vi "Determine Active DTCs and Timestamps.vi"(9 "current time":timestamp, 10 "Previous Changed DTCs":T2[](array[typedef]), 11 "current DTCs":T1[](array[typedef])) -> (3 "Active DTCs":T2[](array[typedef]))   [LabVIEW 2015, in "Diagnostics Addon Engine.lvlib"]
doc: "Does this:\n- if DTC is no longer active, delete it\n- if DTC is new, add it, if it has been there before, update it to latest data\n- Sort DTCs - newest first"
uses:
  Diagnostics Addon Engine.lvlib
  Shared/Types/DTC.Info.ctl
  <vilib>/Automotive Diagnostic Command Set/Diagnostic Protocols.llb/Diagnostic Trouble Code.ctl
  Shared/Diagnostics Addon Shared.lvlib
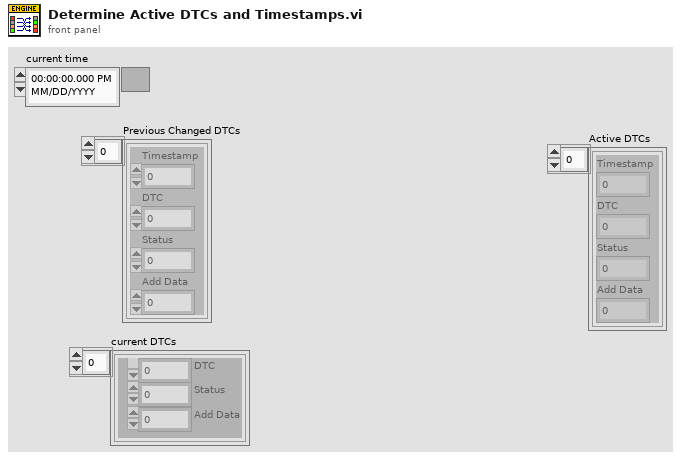
[diagram p1: front panel]
types:
  T1 = typedef "Diagnostic Trouble Code.ctl" = cluster{"DTC":u32, "Status":u32, "Add Data":u32}
  T2 = typedef "Diagnostics Addon Shared.lvlib/DTC.Info.ctl" = cluster{"Timestamp":dbl, "DTC":dbl, "Status":dbl, "Add Data":dbl}
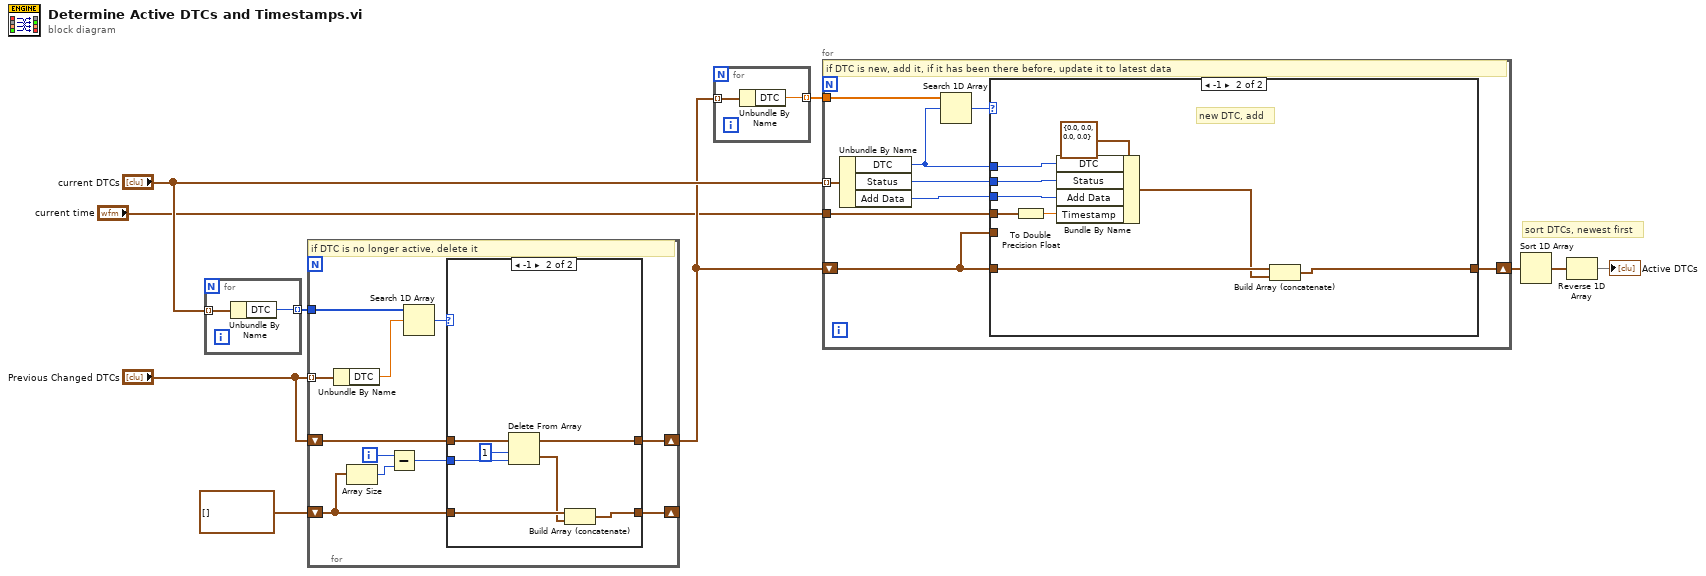
[diagram p0: block diagram]
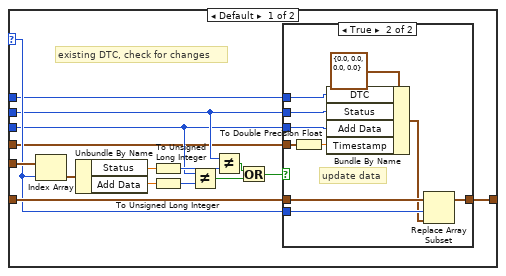
[diagram p3: hidden frame]
diagram:
  # "sort DTCs, newest first"
  n1 = for {
    tunnel: "current DTCs" -> [w12] mode=indexing
    tunnel: [w11] -> w8 mode=indexing
    n2 = Unbundle By Name(w12) -> ("DTC"=w11:u32)
  }
  n3 = for {
    tunnel: "Previous Changed DTCs" -> [w21] mode=indexing
    tunnel: w8 -> [w23]
    shift-right: [w19] -> w3
    shift-left: "Previous Changed DTCs" -> [w20]
    shift-right: [w16] -> _
    shift-left: T2[] [] ("Previous Changed DTCs") -> [w15]
    i -> [w17]
    # "if DTC is no longer active, delete it"
    n4 = Unbundle By Name(w21) -> ("DTC"=w18:dbl)
    n5 = Array Size(array=w15) -> (size(s)=w13:i32)
    n6 = Subtract(x=w17, y=w13) -> (x-y=w14:i32)
    n7 = Search 1D Array(1D array=w23, element=w18) -> (index of element=w22:i32)  [unwired: 1 in]
    n8 = case shown="-1" w22 {
      tunnel: w20 -> [w25 w32]
      tunnel: [w25 w31] -> w19
      tunnel: w14 -> [_ w30]
      tunnel: [w24 w26] -> w16
      tunnel: w15 -> [w24 w28]
      frame Default {
      }
      frame -1 {
        n9 = Delete From Array(array=w32, length=1, index=w30) -> (deleted portion=w27:T2[], array with subset deleted=w31:T2[])
        n10 = Build Array (concatenate)(w28, w27) -> (w26:T2[])
      }
    }
  }
  n11 = for {
    tunnel: w3 -> [w34] mode=indexing
    tunnel: [w33] -> w9 mode=indexing
    n12 = Unbundle By Name(w34) -> ("DTC"=w33:dbl)
  }
  n13 = for {
    tunnel: "current DTCs" -> [w41] mode=indexing
    tunnel: w9 -> [w43]
    shift-right: [w40] -> w2
    shift-left: w3 -> [w35]
    tunnel: "current time" -> [w39]
    # "if DTC is new, add it, if it has been there before, update it to latest data"
    n14 = Unbundle By Name(w41) -> ("DTC"=w37:u32, "Status"=w38:u32, "Add Data"=w36:u32)
    n15 = Search 1D Array(1D array=w43, element=w37) -> (index of element=w42:i32)  [unwired: 1 in]
    n16 = case shown="-1" w42 {
      selector: w42 -> [w49 _]
      tunnel: w35 -> [w50 w79]
      tunnel: [w48 w78] -> w40
      tunnel: w39 -> [w44 w73]
      tunnel: w38 -> [w46 w76]
      tunnel: w37 -> [w47 w75]
      tunnel: w36 -> [w45 w74]
      tunnel: w35 -> [w59 _]
      frame Default {
        # "existing DTC, check for changes"
        n17 = Index Array(array=w59, index=w49) -> (element=w58:T2)
        n18 = Unbundle By Name(w58) -> ("Status"=w57:dbl, "Add Data"=w56:dbl)
        n19 = To Unsigned Long Integer(number=w57) -> (unsigned 32bit integer=w55:u32)
        n20 = To Unsigned Long Integer(number=w56) -> (unsigned 32bit integer=w54:u32)
        n21 = Not Equal?(x=w45, y=w54) -> (x != y?=w53:bool)
        n22 = Not Equal?(x=w46, y=w55) -> (x != y?=w52:bool)
        n23 = Or(x=w52, y=w53) -> (x .or. y?=w51:bool)
        n24 = case shown="True" w51 {
          tunnel: w50 -> [w60 w70]
          tunnel: w49 -> [_ w69]
          tunnel: [w60 w61] -> w48
          tunnel: w47 -> [_ w66]
          tunnel: w46 -> [_ w65]
          tunnel: w45 -> [_ w64]
          tunnel: w44 -> [_ w63]
          frame False {
          }
          frame True {
            # "update data"
            n25 = To Double Precision Float(number=w63) -> (double precision float=w68:dbl)
            n26 = Bundle By Name(cluster=T2 {"Timestamp"=0.0, "DTC"=0.0, "Status"=0.0, "Add Data"=0.0} ("Diagnostic Trouble Code"), "DTC"=w66, "Status"=w65, "Add Data"=w64, "Timestamp"=w68) -> (w62:T2)
            n27 = Replace Array Subset(array=w70, new element=w62, index=w69) -> (w61:T2[])
          }
        }
      }
      frame -1 {
        # "new DTC, add"
        n28 = To Double Precision Float(number=w73) -> (double precision float=w72:dbl)
        n29 = Bundle By Name(cluster=T2 {"Timestamp"=0.0, "DTC"=0.0, "Status"=0.0, "Add Data"=0.0} ("Diagnostic Trouble Code"), "DTC"=w75, "Status"=w76, "Add Data"=w74, "Timestamp"=w72) -> (w71:T2)
        n30 = Build Array (concatenate)(w79, w71) -> (w78:T2[])
      }
    }
  }
  n31 = Sort 1D Array(array=w2) -> (sorted array=w5:T2[])
  n32 = Reverse 1D Array(array=w5) -> (reversed array=→"Active DTCs":T2[])
